vi "UUDT Engine Connection List.vi"(7 "Action":T1, 8 "error in":errorcluster, 10 "Queue List":refnum<queue>[](array[refnum]), 11 "UUDT":u32) -> (0 "error out":errorcluster, 2 "Queue List":refnum<queue>[](array[refnum]))   [LabVIEW 2019, in "GMLAN.lvlib"]
uses:
  GMLAN.lvlib
  _Types/UUDT Engine Connection List_Action.ctl
  _Types/UUDT Messages.ctl
  _Types/UUDT Responses.ctl
  <vilib>/xnet/xnet.llb/XNET Frame CAN.ctl
  <vilib>/xnet/xnet.llb/XNET Frame Type CAN.ctl
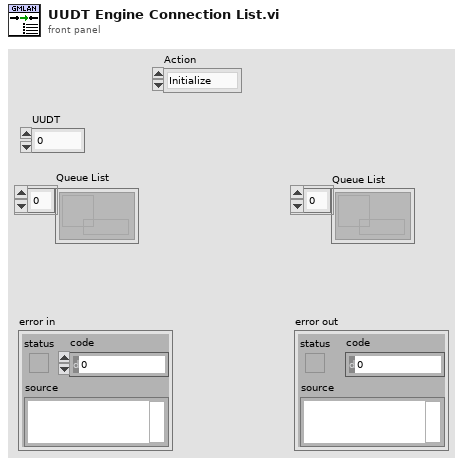
[diagram p1: front panel]
types:
  T1 = typedef "GMLAN.lvlib/UUDT Engine Connection List_Action.ctl" = enum8{"Initialize", "Write", "Add", "Read"}
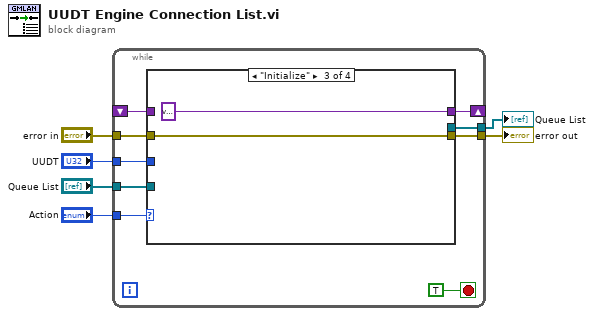
[diagram p0: block diagram]
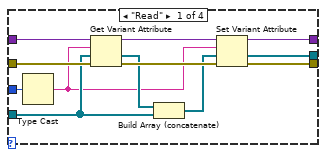
[diagram p2: hidden frame]
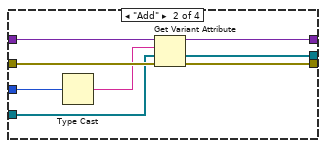
[diagram p3: hidden frame]
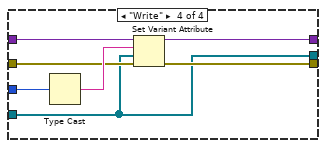
[diagram p4: hidden frame]
diagram:
  n1 = while {
    shift-right: [w13] -> _
    shift-left: _ -> [w14]
    tunnel: "UUDT" -> [w15]
    tunnel: "error in" -> [w12]
    tunnel: [w11] -> w5
    tunnel: "Action" -> [w9]
    tunnel: "Queue List" -> [w8]
    tunnel: [w7] -> w1
    stop <- TRUE stop-if-true
    n2 = case shown="\"Initialize\"" w9 {
      tunnel: w15 -> [w24 w32 _ w43]
      tunnel: w14 -> [w25 w33 _ w41]
      tunnel: [w20 w29 variant ("variant") w40] -> w13
      tunnel: w12 -> [w26 w34 w36 w39]
      tunnel: [w22 w30 w36 w38] -> w11
      tunnel: w8 -> [w18 w28 _ w37]
      tunnel: [w16 w27 _ w37] -> w7
      frame "Read" {
        n3 = Type Cast(x=w24) -> (*(type *) &x=w17:string)  [unwired: 1 in]
        n4 = Get Variant Attribute(Variant=w25, name=w17, default value (empty Variant)=w18, error in=w26) -> (duplicate Variant=w21:variant, value=w19:refnum<queue>[], error out=w23:errorcluster)  [unwired: 1 out]
        n5 = Build Array (concatenate)(w19, w18) -> (w16:refnum<queue>[])
        n6 = Set Variant Attribute(Variant=w21, name=w17, value=w16, error in=w23) -> (Variant out=w20:variant, error out=w22:errorcluster)  [unwired: 1 out]
      }
      frame "Add" {
        n7 = Type Cast(x=w32) -> (*(type *) &x=w31:string)  [unwired: 1 in]
        n8 = Get Variant Attribute(Variant=w33, name=w31, default value (empty Variant)=w28, error in=w34) -> (duplicate Variant=w29:variant, value=w27:refnum<queue>[], error out=w30:errorcluster)  [unwired: 1 out]
      }
      frame "Initialize" {
      }
      frame "Write" {
        n9 = Type Cast(x=w43) -> (*(type *) &x=w42:string)  [unwired: 1 in]
        n10 = Set Variant Attribute(Variant=w41, name=w42, value=w37, error in=w39) -> (Variant out=w40:variant, error out=w38:errorcluster)  [unwired: 1 out]
      }
    }
  }
  "error out" <- w5
  "Queue List" <- w1
